vi "Set LabVIEW Array Parameter by expression.vi"(0 "QPA Measurement in":refnum<class "QPA Measurement.lvclass">, 5 "Step In":refnum<k7>, 7 "LabVIEW Parameter to Set":string, 9 "Array of Expresssions":string[](array[string]), 11 "error in (no error)":errorcluster) -> (4 "QPA Measurement out":refnum<class "QPA Measurement.lvclass">, 6 "Step Out":refnum<k7>, 15 "error out":errorcluster)   [LabVIEW 2016, in "QPA Measurement.lvlib" / "QPA Measurement.lvclass"]
uses:
  QPA Measurement.lvclass
  C:/Projects/STS/Common/Sequence Automation/Plugins/Measurement Interface.lvlibp/Measurement Interface.lvclass
  Plugins/Measurement Interface.lvlibp/Private Methods/Engine Reference/Read Engine Reference.vi
  Plugins/TestStand API Tools (TSAT).lvlibp/Step Actions/TSAT Step Actions.lvlib
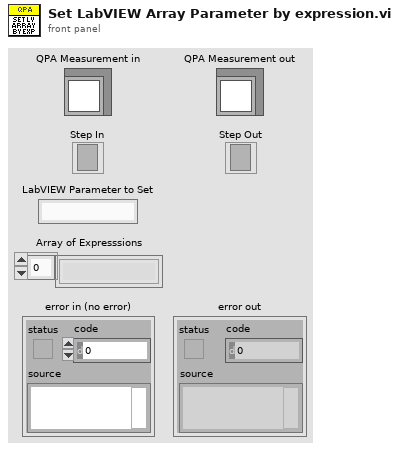
[diagram p1: front panel]
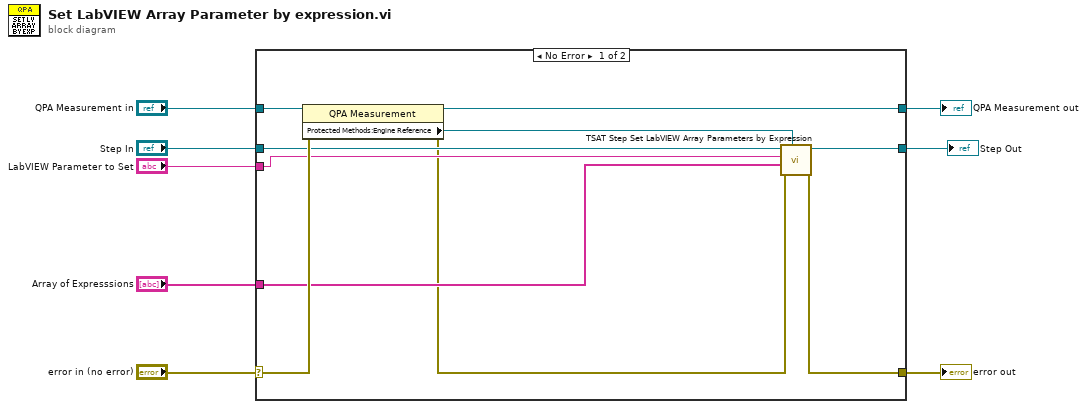
[diagram p0: block diagram]
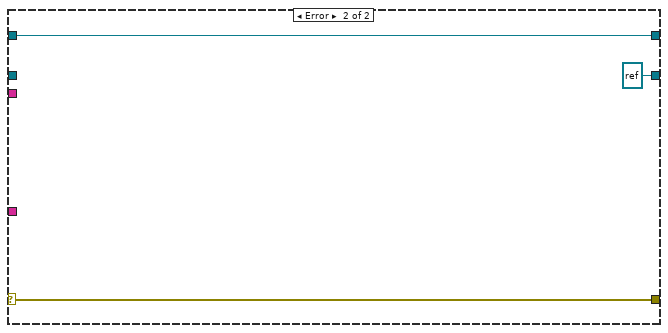
[diagram p2: hidden frame]
diagram:
  n1 = case shown="No Error" "error in (no error)" {
    selector: "error in (no error)" -> [w18 w21]
    tunnel: [w17 w21] -> w7
    tunnel: [w10 w20] -> w5
    tunnel: "QPA Measurement in" -> [w11 w20]
    tunnel: "Array of Expresssions" -> [w16 _]
    tunnel: "LabVIEW Parameter to Set" -> [w13 _]
    tunnel: "Step In" -> [w15 _]
    tunnel: [w14 refnum<k7> refnum ("Step Out")] -> w2
    frame No Error {
      n2 = property class="QPA Measurement"(reference=w11, error in=w18) -> (reference out=w10:refnum<class "QPA Measurement.lvclass">, error out=w12:errorcluster, "Protected Methods:Engine Reference"=w9:refnum<k7>)
      n3 = call "TSAT Step Set LabVIEW Array Parameters by Expression.vi"("Engine In"=w9, "Error In"=w12, "Value Expressions"=w16, "Parameter to Set"=w13, "Step In"=w15) -> ("Error Out"=w17:errorcluster, "Step Out"=w14:refnum<k7>)  [unwired: 5 in]
    }
    frame Error {
    }
  }
  "error out" <- w7
  "QPA Measurement out" <- w5
  "Step Out" <- w2
